vi "receive message.vi"(8 "error in (no error)":errorcluster, 11 "Socket in":refnum<class "Socket.lvclass">) -> (0 "error out":errorcluster, 3 "Socket out":refnum<class "Socket.lvclass">)   [LabVIEW 2018, in "Socket.lvclass"]
uses:
  Socket.lvclass
  Socket.lvclass/Socket.ctl
  <vilib>/addons/zeromq/zmq_socket.lvclass
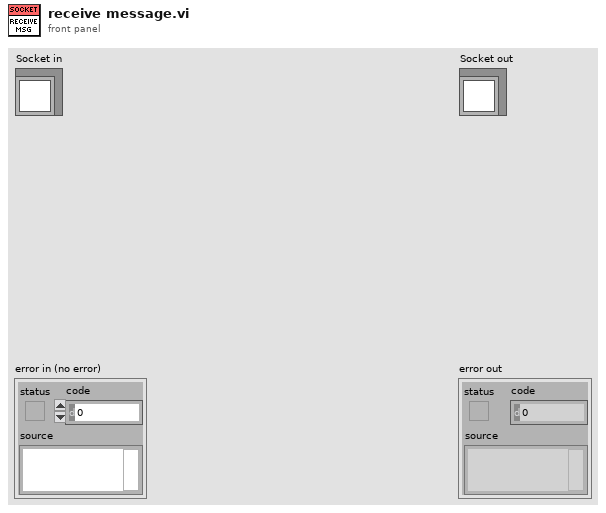
[diagram p1: front panel]
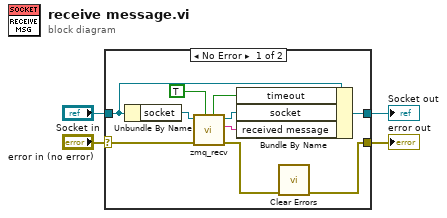
[diagram p0: block diagram]
diagram:
  n1 = case shown="No Error" "error in (no error)" {
    selector: "error in (no error)" -> [w14 w16]
    tunnel: [w6 w16] -> w3
    tunnel: [w11 w15] -> w1
    tunnel: "Socket in" -> [w12 w15]
    frame No Error {
      n2 = Unbundle By Name(w12) -> ("socket"=w13:refnum<class "zmq_socket.lvclass">)
      n3 = call <vilib>:"zmq_recv.vi"("no block? (F)"=TRUE, "error in"=w14, "socket in"=w13) -> ("error out"=w7:errorcluster, "data"=w9:string, "socket out"=w10:refnum<class "zmq_socket.lvclass">, "timeout?"=w8:bool)  [unwired: 2 in, 1 out]
      n4 = Bundle By Name(cluster=w12, "timeout"=w8, "socket"=w10, "received message"=w9) -> (w11:refnum<class "Socket.lvclass">)
      n5 = call <vilib>:"Clear Errors.vi"("error in (no error)"=w7) -> ("error out"=w6:errorcluster)  [unwired: 5 in, 1 out]
    }
    frame Error {
    }
  }
  "error out" <- w3
  "Socket out" <- w1
